vi "Log Sleep.vi"(8 "error in (no error)":errorcluster, 10 "String":string, 11 "Cluster in":T1) -> (0 "error out":errorcluster, 3 "Cluster out":T1)   [LabVIEW 2019]
doc: "Incorporate guard log entries into both maps contained within the Day 4 cluster data."
uses:
  Log Entry.ctl
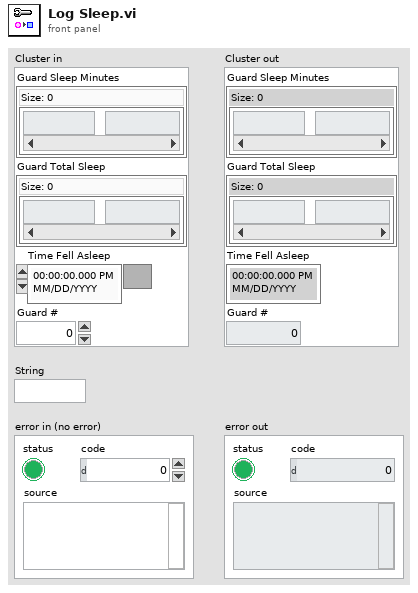
[diagram p1: front panel]
types:
  T1 = typedef "Log Entry.ctl" = cluster{"Guard Sleep Minutes":map{string, i32}, "Guard Total Sleep":map{string, i32}, "Time Fell Asleep":timestamp, "Guard #":i32}
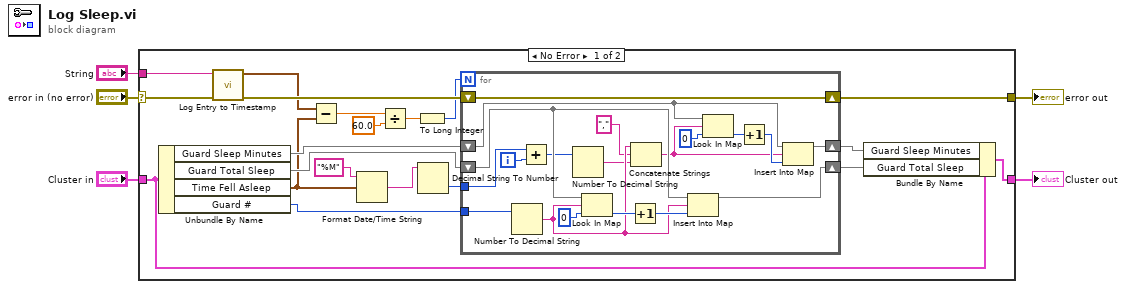
[diagram p0: block diagram]
diagram:
  n1 = case shown="No Error" "error in (no error)" {
    selector: "error in (no error)" -> [w6 w46]
    tunnel: "Cluster in" -> [w21 w45]
    tunnel: [w20 w45] -> w4
    tunnel: [w14 w46] -> w3
    tunnel: "String" -> [w7 _]
    frame No Error {
      n2 = Unbundle By Name(w21) -> ("Guard Sleep Minutes"=w24:map{string, i32}, "Guard Total Sleep"=w25:map{string, i32}, "Time Fell Asleep"=w22:timestamp, "Guard #"=w23:i32)
      n3 = call "Log Entry to Timestamp.vi"("error in (no error)"=w6, "String"=w7) -> ("error out"=w13:errorcluster, "Time Stamp"=w8:timestamp)  [unwired: 8 in]
      n4 = Subtract(x=w8, y=w22) -> (x-y=w10:dbl)
      n5 = Format Date/Time String(time format string (%c)="%M", seconds (now)=w22) -> (date/time string=w16:string)  [unwired: 1 in]
      n6 = Divide(x=w10, y=60.0) -> (x/y=w9:dbl)
      n7 = To Long Integer(number=w9) -> (32bit integer=w12:i32)
      n8 = Decimal String To Number(string=w16) -> (number=w17:i32)  [unwired: 2 in, 1 out]
      n9 = for {
        N: w12 -> [_]
        tunnel: w23 -> [w44]
        shift-right: [w42] -> w14
        shift-left: w13 -> [w42]
        shift-right: [w38] -> w19
        shift-left: w25 -> [w41]
        shift-right: [w26] -> w18
        shift-left: w24 -> [w27]
        tunnel: w17 -> [w33]
        i -> [w34]
        n10 = Number To Decimal String(number=w44) -> (decimal integer string=w37:string)  [unwired: 1 in]
        n11 = Add(x=w33, y=w34) -> (x+y=w32:i32)
        n12 = Number To Decimal String(number=w32) -> (decimal integer string=w31:string)  [unwired: 1 in]
        n13 = Look In Map(map=w41, key=w37, default value=0) -> (value=w40:i32)  [unwired: 1 out]
        n14 = Increment(x=w40) -> (x+1=w39:i32)
        n15 = Concatenate Strings(w37, "," ("string"), w31) -> (w28:string)
        n16 = Insert Into Map(map in=w41, key=w37, value=w39) -> (map out=w38:map{string, i32})  [unwired: 2 out]
        n17 = Look In Map(map=w27, key=w28, default value=0) -> (value=w30:i32)  [unwired: 1 out]
        n18 = Increment(x=w30) -> (x+1=w29:i32)
        n19 = Insert Into Map(map in=w27, key=w28, value=w29) -> (map out=w26:map{string, i32})  [unwired: 2 out]
      }
      n20 = Bundle By Name(cluster=w21, "Guard Sleep Minutes"=w18, "Guard Total Sleep"=w19) -> (w20:T1)
    }
    frame Error {
    }
  }
  "Cluster out" <- w4
  "error out" <- w3
